vi "Open_File_for_write_check.vi"(8 "advisory dialog? (display:T)":bool=TRUE, 9 "append to file? (new file:F)":bool, 11 "file path":path) -> (0 "error out":errorcluster, 3 "refnum":refnum<file>)   [LabVIEW 2011]
doc: "Opens an existing file, creates a new file, or replaces an existing file, programmatically or interactively using dialog. You can optionally specify a dialog prompt, default file name, start path, or filter pattern, and you can specify open and deny modes when opening a file, plus group and permission when creating a new file. Use this VI with the intermediate Write File+ or Read File+ VIs described below.\n\nfile path is the path name of the file. If file path is empty (default value) or is Not A Path, the VI displays a File dialog box from which you can select a file. Error 43 occurs if the user cancels the dialog. \n\nfunction is the operation to perform:\n\n 0 (open) opens an existing file. Error 7 occurs if the file cannot be found.\n \n 1 (open or create) opens an existing file or creates a new file if one does not exist.\n\n 2 (create or replace) creates a new file or replaces a file if it exists and you give permission. Replacement is done by opening the file and setting EOF to 0. Error 43 occurs if the user elects to disallow the replacement using dialog. \n\n 3 (create) creates a new file. Error 8 occurs if the file already exists.\n\nadvisory dialog? Set TRUE (default) if you want a dialog if function=0 and the file does not exist, or if function=2 or 3 and the file exists.\n\nprompt is the message that appears below the list of files and directories in the file dialog.\n\ndefault name is the initial file name that appears in the selection box of the file dialog.\n\nstart path is the path name to the initially displayed directory in a file dialog. The default value is Not A Path, which is the path to the last directory shown in a file dialog.\n\npattern is the match pattern specification to display only certain types of files or directories. See the description of the File Dialog function for more information.\n\nerror in is a cluster of three elements (error?, code, and source) that describe the upstream error state, that is, the existance of any error preceeding the execution of the VI. The VI executes normally only if no incoming error exists; otherwise it merely passes the error in value to error out. error? is TRUE if an error occurred; the default value is FALSE. code is the error code; the default value is 0. source is in most cases the name of the VI or function that produced the error; the default value is an empty string.\n\nnew file path is the path of the file opened or created. You can use this output to determine the path of a file that you open or create using dialog. new file path returns Not A Path if the user selects Cancel from the dialog box.\n\nrefnum is the reference number of the open file. The value is Not A Refnum if the file cannot be opened.\n\nfile size is the size of the file in bytes; it is also the location of the end of file.\n\nerror out is a cluster of three elements (error?, code, and source) that describe the error state following the execution of the VI. If an incoming error does not exist, the VI executes normally and error out describes the VI's error state; if an incoming error exists, error out equals error in."
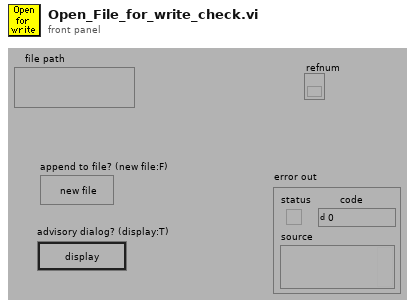
[diagram p1: front panel]
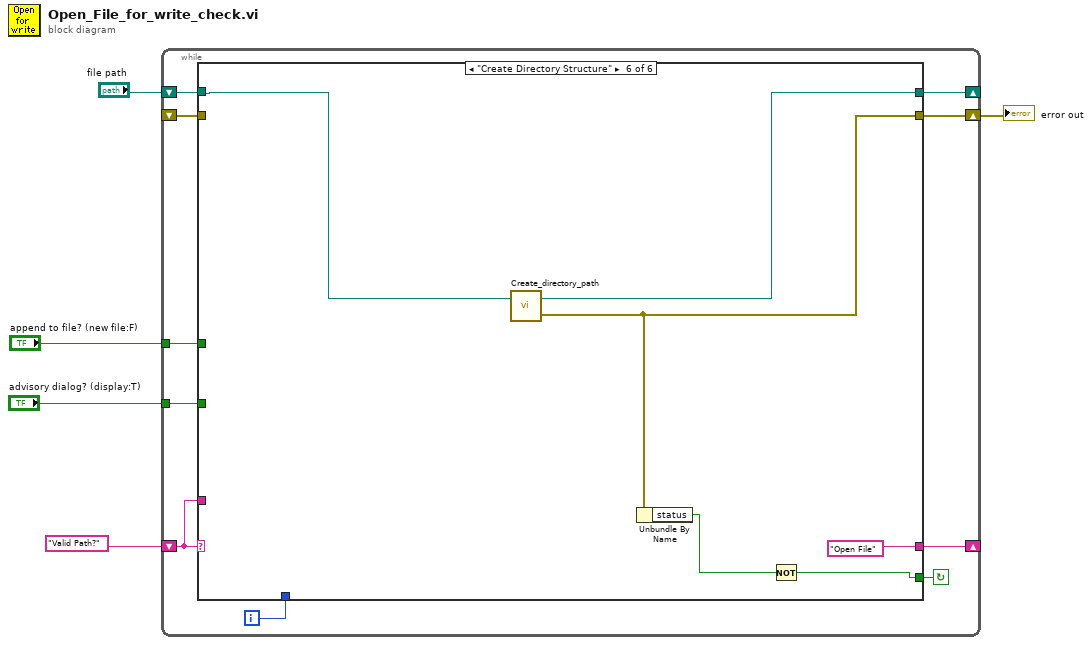
[diagram p0: block diagram]
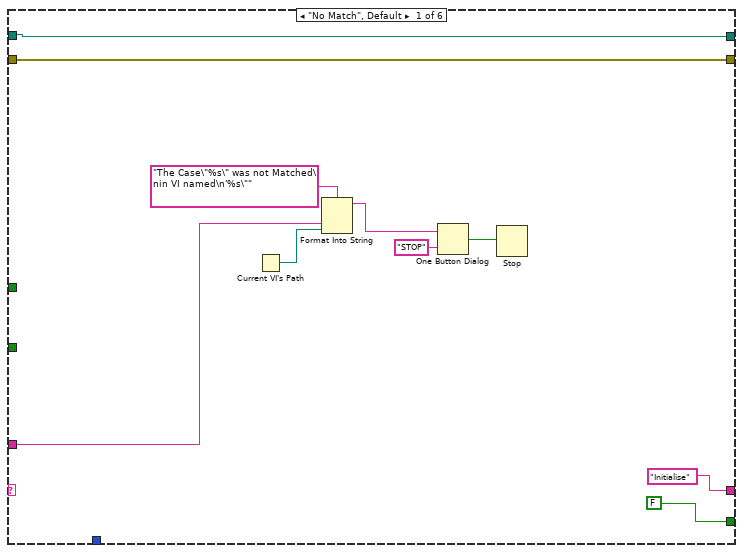
[diagram p2: hidden frame]
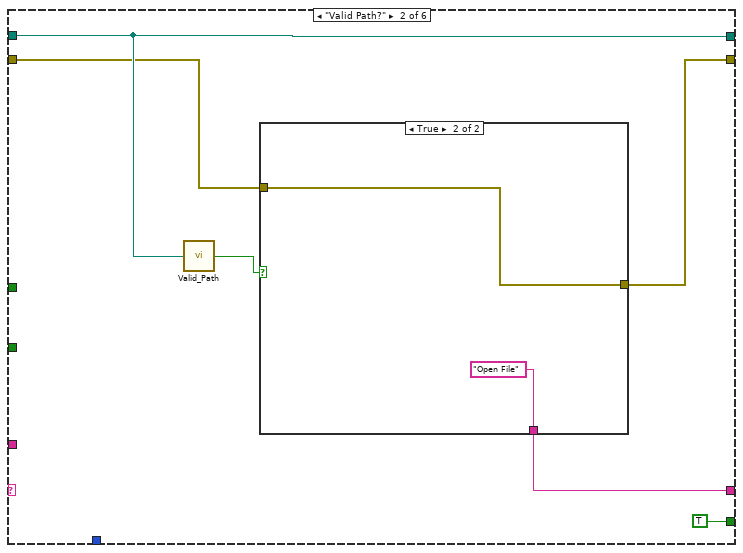
[diagram p3: hidden frame]
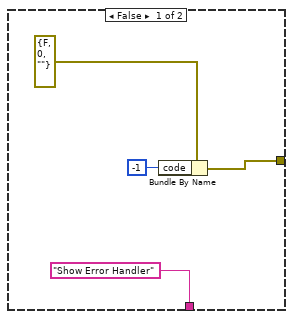
[diagram p4: hidden frame]
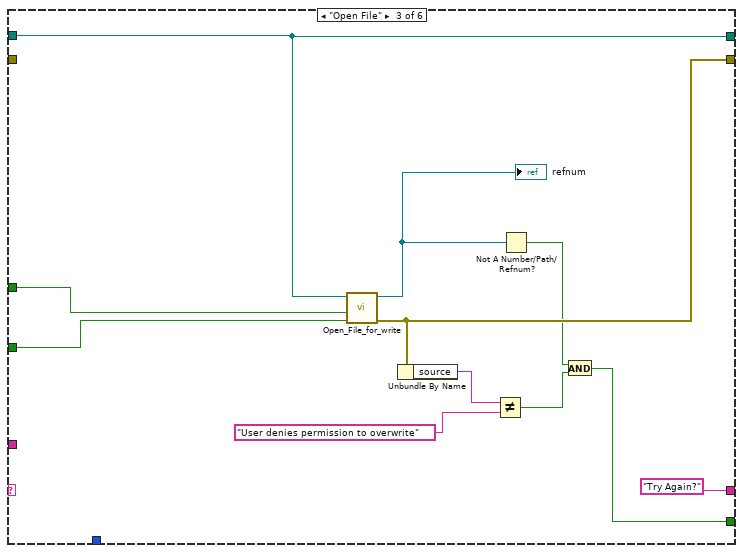
[diagram p5: hidden frame]
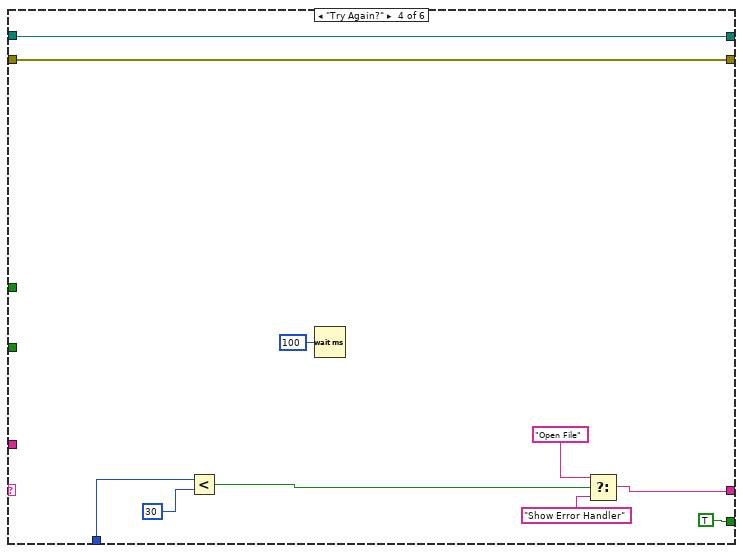
[diagram p6: hidden frame]
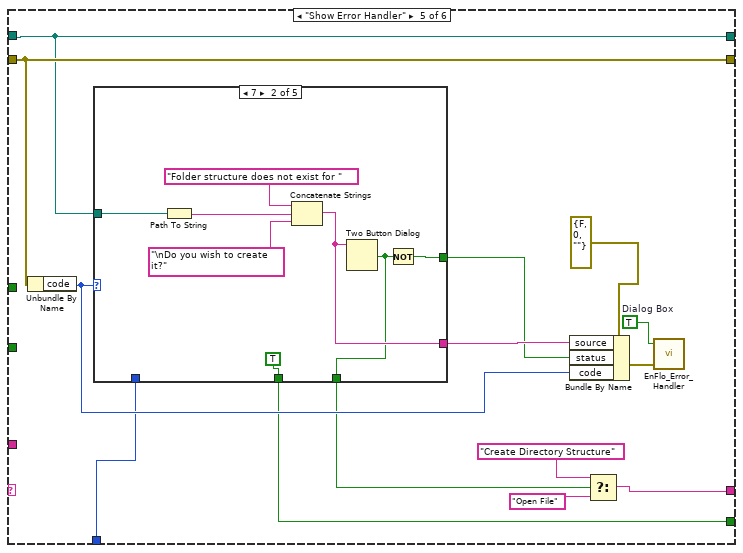
[diagram p7: hidden frame]
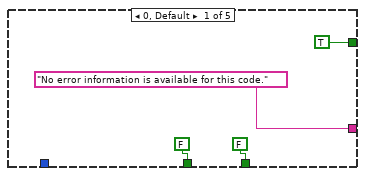
[diagram p8: hidden frame]
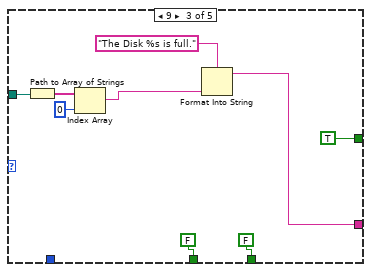
[diagram p9: hidden frame]
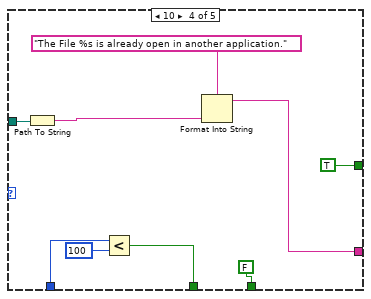
[diagram p10: hidden frame]
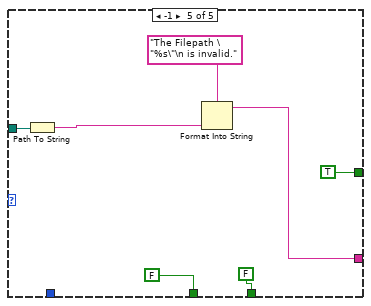
[diagram p11: hidden frame]
diagram:
  n1 = while {
    shift-left: "Valid Path?" -> [w13]
    shift-right: [w14] -> _
    tunnel: "append to file? (new file:F)" -> [w12]
    tunnel: "advisory dialog? (display:T)" -> [w11]
    shift-right: [w9] -> w2
    shift-left: _ -> [w6]
    shift-right: [w7] -> _
    shift-left: "file path" -> [w8]
    i -> [w10]
    stop <- w15 continue-if-true
    n2 = case shown="\"Create Directory Structure\"" w13 {
      tunnel: [FALSE TRUE w38 TRUE w60 w112] -> w15
      tunnel: ["Initialise" w29 "Try Again?" w53 w72 "Open File"] -> w14
      tunnel: w13 -> [w20 _ _ _ _ _]
      tunnel: w12 -> [_ _ w47 _ _ _]
      tunnel: w11 -> [_ _ w46 _ _ _]
      tunnel: w8 -> [w17 w31 w44 w49 w68 w114]
      tunnel: w10 -> [_ _ _ w56 w59 _]
      tunnel: [w16 w27 w43 w50 w69 w110] -> w9
      tunnel: [w17 w31 w44 w49 w68 w115] -> w7
      tunnel: w6 -> [w16 w26 _ w50 w69 _]
      frame "No Match", Default {
        n3 = Current VI's Path() -> (path=w19:path)
        n4 = Format Into String(format string="The Case\"%s\" was not Matched\nin VI named\n'%s\"" ("Format String"), w20, w19) -> (resulting string=w23:string)  [unwired: 2 in, 1 out]
        n5 = One Button Dialog(message=w23, button name ("OK")="STOP") -> (true=w21:bool)
        n6 = Stop(stop? (T)=w21) -> ()
      }
      frame "Valid Path?" {
        n7 = call "Valid_Path.vi"("Filename"=w31) -> ("Valid Path?"=w30:bool)
        n8 = case shown="True" w30 {
          tunnel: ["Show Error Handler" "Open File"] -> w29
          tunnel: [w34 w36] -> w27
          tunnel: w26 -> [_ w36]
          frame False {
            n9 = Bundle By Name(cluster=errorcluster {"status"=FALSE, "code"=0, "source"=""} ("error in (no error)"), "code"=-1) -> (w34:errorcluster)
          }
          frame True {
          }
        }
      }
      frame "Open File" {
        n10 = call "Open_File_for_write.vi"("advisory dialog? (display:T)"=w46, "append to file? (new file:F)"=w47, "file path"=w44) -> ("error out"=w43:errorcluster, "refnum"=w45:refnum<file>)  [unwired: 7 out]
        "refnum" <- w45
        n11 = Unbundle By Name(w43) -> ("source"=w41:string)
        n12 = Not Equal?(x=w41, y="User denies permission to overwrite") -> (x != y?=w40:bool)
        n13 = Not A Number/Path/Refnum?(number/path/refnum=w45) -> (NaN/Path/Refnum?=w39:bool)
        n14 = And(x=w39, y=w40) -> (x .and. y?=w38:bool)
      }
      frame "Try Again?" {
        n15 = Less?(x=w56, y=30) -> (x < y?=w54:bool)
        n16 = Wait (ms)(milliseconds to wait=u32 100) -> ()  [unwired: 1 out]
        n17 = Select(t="Open File", s=w54, f="Show Error Handler") -> (s? t:f=w53:string)
      }
      frame "Show Error Handler" {
        w67 = TRUE  # Dialog Box
        n18 = Unbundle By Name(w69) -> ("code"=w63:i32)
        n19 = case shown="7" w63 {
          tunnel: w68 -> [_ w81 w93 w102 w109]
          tunnel: ["No error information is available for this code." w80 w88 w100 w107] -> w64
          tunnel: [FALSE w78 FALSE FALSE FALSE] -> w62
          tunnel: [TRUE w79 TRUE TRUE TRUE] -> w61
          tunnel: [FALSE TRUE FALSE w94 FALSE] -> w60
          tunnel: w59 -> [_ _ _ w96 _]
          frame 0, Default {
          }
          frame 7 {
            n20 = Path To String(path=w81) -> (string=w83:string)
            n21 = Concatenate Strings("Folder structure does not exist for ", w83, "\nDo you wish to create it?") -> (w80:string)
            n22 = Two Button Dialog(message=w80) -> (T button?=w78:bool)  [unwired: 2 out]
            n23 = Not(x=w78) -> (.not. x?=w79:bool)
          }
          frame 9 {
            n24 = Path to Array of Strings(0:w93) -> (2:w92:string[])  [unwired: 1 out]
            n25 = Index Array(array=w92, index=0 ("Index")) -> (element=w90:string)
            n26 = Format Into String(format string="The Disk %s is full." ("Format String"), w90) -> (resulting string=w88:string)  [unwired: 2 in, 1 out]
          }
          frame 10 {
            n27 = Path To String(path=w102) -> (string=w99:string)
            n28 = Less?(x=w96, y=100) -> (x < y?=w94:bool)
            n29 = Format Into String(format string="The File %s is already open in another application." ("Format String"), w99) -> (resulting string=w100:string)  [unwired: 2 in, 1 out]
          }
          frame -1 {
            n30 = Path To String(path=w109) -> (string=w106:string)
            n31 = Format Into String(format string="The Filepath \"%s\"\n is invalid." ("Format String"), w106) -> (resulting string=w107:string)  [unwired: 2 in, 1 out]
          }
        }
        n32 = Bundle By Name(cluster=errorcluster {"status"=FALSE, "code"=0, "source"=""} ("error in (no error)"), "source"=w64, "status"=w61, "code"=w63) -> (w66:errorcluster)
        n33 = Select(t="Create Directory Structure", s=w62, f="Open File") -> (s? t:f=w72:string)
        n34 = call "EnFlo_Error_Handler.vi"("error in (no error)"=w66, "Dialog Box (T)"=w67) -> ()  [unwired: 1 in, 3 out]
      }
      frame "Create Directory Structure" {
        n35 = call "Create_directory_path.vi"("Path name"=w114) -> ("error out"=w110:errorcluster, "Path name Out"=w115:path)  [unwired: 1 in]
        n36 = Unbundle By Name(w110) -> ("status"=w111:bool)
        n37 = Not(x=w111) -> (.not. x?=w112:bool)
      }
    }
  }
  "error out" <- w2
